vi "PixeLink MonitorAndSave.vi"(7 "Racine chemin de sauvegarde":path=path "G:/Développement de Programmes/Programmes/octo-labview/PixeLink - Homebrew/Data") -> ()   [LabVIEW 2014]
uses:
  <vilib>/addons/PixeLINK/Low Level Functions/ACQUISITION.llb/TDPU-Acquisition-StreamState.ctl
  <vilib>/addons/PixeLINK/Low Level Functions/CAMERA_FEATURES.llb/TDPU-CameraFeatures-FeatureIds.ctl
  <vilib>/addons/PixeLINK/Low Level Functions/CAMERA_FEATURES.llb/TDPU-CameraFeatures-FeatureFlags.ctl
  <vilib>/Platform/TimedLoop/XDataNode/timing_clust.ctl
  <vilib>/Platform/TimedLoop/XDataNode/nitl_modes.ctl
  <vilib>/Platform/TimedLoop/XDataNode/wakeup.ctl
  <vilib>/platform/TimedLoop/XDataNode/XDataNode.xnode
  <vilib>/Platform/TimedLoop/XDataNode/XDNodeRunTimeDep.lvlib
panel:
  out "Div":dbl
  out "Imager Serial #":u32[](array[numeric])
  in  "Chemins de sauvegarde":path[](array[path])
  in  "Bind Path to Camera":bool
  in  "Automatic\nfolder naming":bool=TRUE
  in  "Imager":u32(ring)=741003962 items=["Cam 0"=741003962]
  out "Error OUT 2":errorcluster
  out "Error OUT":errorcluster
  in  "Overwrite?":bool
  in  "Snap current Data":bool
  in  "Save Data":bool
  out "Warning":bool
  out "Message":string
  in  "Indice":u32
  in  "Nom du fichier":string="tir"
  in  "Mode de Sauvegarde":u16(ring)=1 items=["Manuel", "Automatique"]
  out "Captured Image":dbl[][](graph)
  out "Waiting for Trigger":bool
  in  "Continuous Grab":bool
  in  "Snap Next frame":bool
  out "Camera Handle":u32
  in  "Stop Grab\n(Insistez!)":bool
  in  "Trigger Type":enum16{"Free Running", "Software", "Hardware"}(ring)
  in  "Trigger Polarity":enum16{"Positive", "Negative"}(ring)
  in  "Refresh Trigger":bool
  in  "Exposure Time":dbl(slide) min=3.9999998989515007e-05 max=1.0 scale=3.9999998989515007e-05..1.0
  in  "stop":bool
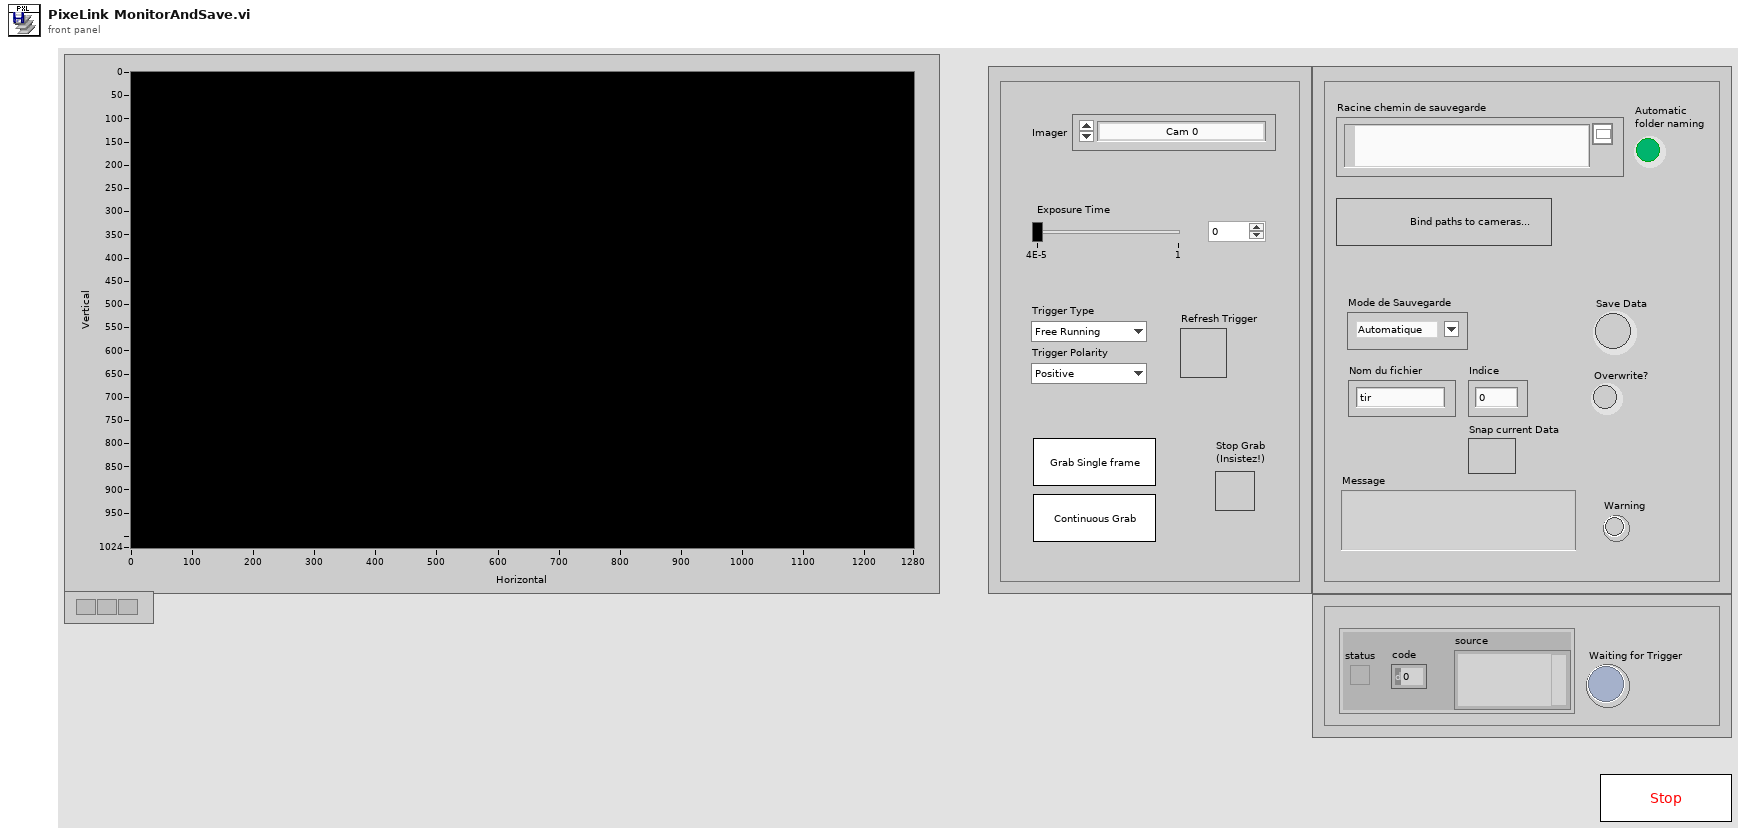
[diagram p1: front panel]
types:
  T1 = typedef "TDPU-Acquisition-StreamState.ctl" = u32
  T2 = typedef "TDPU-CameraFeatures-FeatureFlags.ctl" = u32
  T3 = typedef "TDPU-CameraFeatures-FeatureIds.ctl" = u32
  T4 = typedef "XDNodeRunTimeDep.lvlib/timing_clust.ctl" = cluster{"Expected End [f-1]":u64, "Actual End [f-1]":u64, "Finished Late? [f-1]":bool, "Expected End [i-1]":u64, "Actual End [i-1]":u64, "Finished Late? [i-1]":bool, "Expected Start [i]":u64, "Actual Start [i]":u64, "Expected Start [f]":u64, "Actual Start [f]":u64, "Source Name":string, "Structure Name":string, "Period":i64, "Deadline":i64, "Offset":i64, "Start":i64, "Priority":i32, "Timeout":i32, "Mode":T5, "Wakeup Reason":T6, "Error":errorcluster, "Source Type":string, "Secondary Source Type":string, "Global End Time":u64, "Global Start Time":u64, "Frame Duration":u64, "Iteration Duration":u64, "Assigned CPU":i32, "I/O Scan Engine Mode":u32}
  T5 = typedef "XDNodeRunTimeDep.lvlib/nitl_modes.ctl" = enum32{"No Change", "Process missed periods, maintain original phase", "Discard missed periods, maintain original phase", "Process missed periods, ignore original phase", "Discard missed periods, ignore original phase"}
  T6 = typedef "XDNodeRunTimeDep.lvlib/wakeup.ctl" = enum32{"Normal", "Aborted", "Asynchronous wakeup", "Timing source error", "Timed loop error", "Timeout"}
  T7 = typedef "LVStringsAndValuesArrayTypeDef_U32.ctl" = cluster{"String":string, "Value":u32}[]
  T8 = typedef "TDPU-Identification-Camera_Info.ctl" = cluster{"VendorName":string, "ModelName":string, "Description":string, "SerialNumber":string, "FirmwareVersion":string, "FPGAVersion":string, "CameraName":string}
  T9 = typedef "TDPU-Acquisition-Frame_Desc.ctl" = cluster{"uSize":u32, "fFrameTime":dbl, "uFrameNumber":u32, "Brightness":cluster{"fValue":dbl}, "AutoExposure":cluster{"fValue":dbl}, "Sharpness":cluster{"fValue":dbl}, "WhiteBalance":cluster{"fValue":dbl}, "Hue":cluster{"fValue":dbl}, "Saturation":cluster{"fValue":dbl}, "Gamma":cluster{"fValue":dbl}, "Shutter":cluster{"fValue":dbl}, "Gain":cluster{"fValue":dbl}, "Iris":cluster{"fValue":dbl}, "Focus":cluster{"fValue":dbl}, "Temperature":cluster{"fValue":dbl}, "Trigger":cluster{"fMode":dbl, "fType":dbl, "fPolarity":dbl, "fDelay":dbl, "fParameter":dbl}, "Zoom":cluster{"fValue":dbl}, "Pan":cluster{"fValue":dbl}, "Tilt":cluster{"fValue":dbl}, "OpticalFilter":cluster{"fValue":dbl}, "GPIO":cluster{"fMode":dbl[], "fPolarity":dbl[], "fParameter1":dbl[], "fParameter2":dbl[], "fParameter3":dbl[]}, "FrameRate":cluster{"fValue":dbl}, "ROI":cluster{"fLeft":dbl, "fTop":dbl, "fWidth":dbl, "fHeight":dbl}, "Flip":cluster{"fHorizontal":dbl, "fVertical":dbl}, "PixelAddressingValue":cluster{"fValue":dbl}, "PixelFormat":cluster{"fValue":dbl}, "ExtendedShutter":cluster{"fKneePoint":dbl[]}, "AutoROI":cluster{"fLeft":dbl, "fTop":dbl, "fWidth":dbl, "fHeight":dbl}, "WhiteShading":cluster{"fRedGain":dbl, "fGreenGain":dbl, "fBlueGain":dbl}, "Rotate":cluster{"fValue":dbl}, "PixelAddressingMode":cluster{"fValue":dbl}}
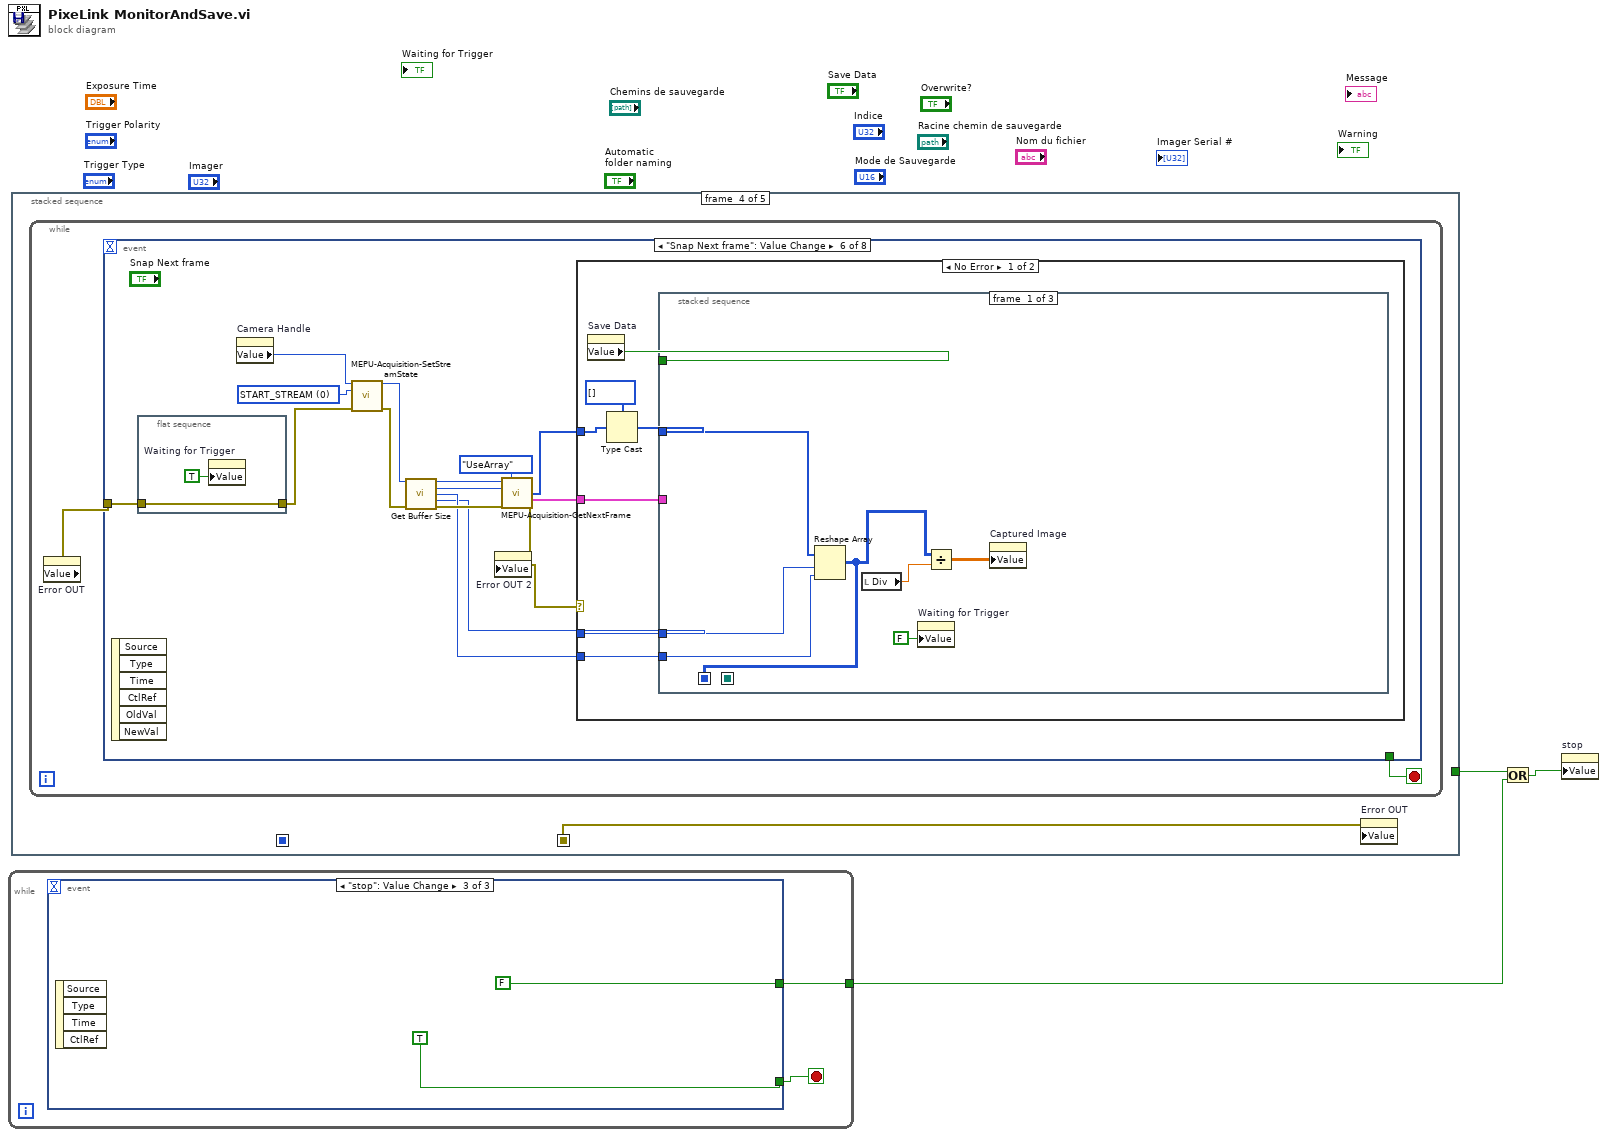
[diagram p0: block diagram]
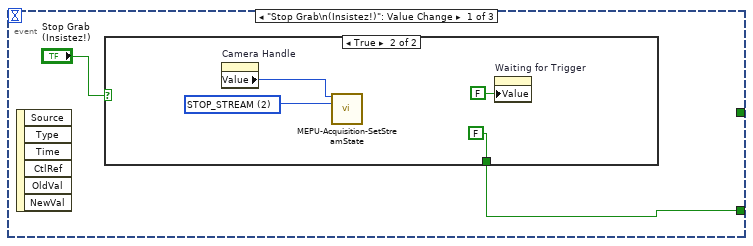
[diagram p2: hidden frame]
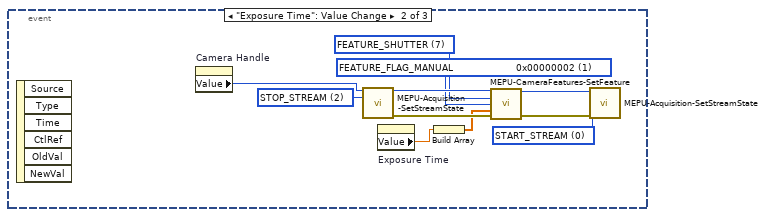
[diagram p4: hidden frame]
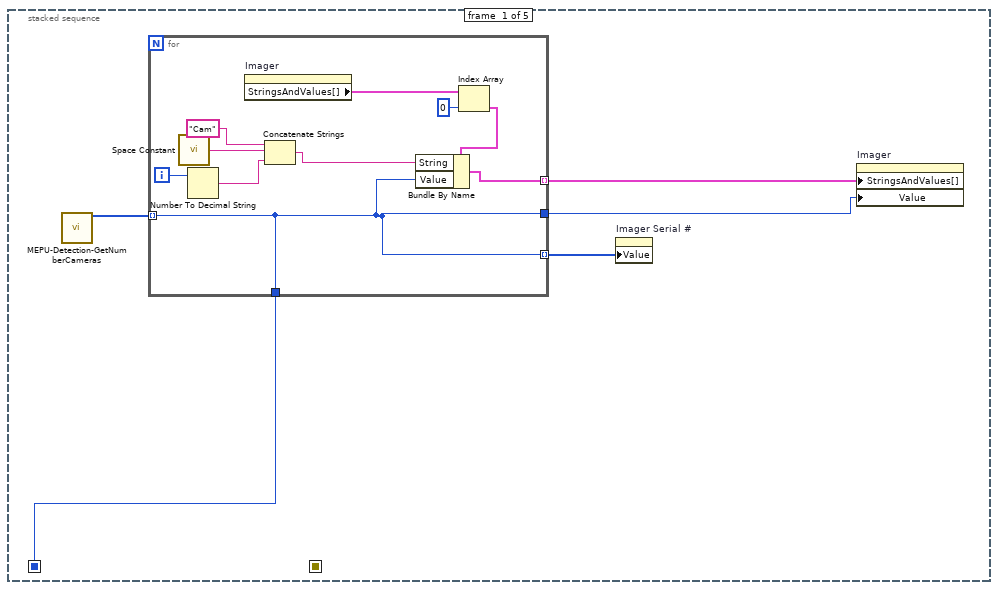
[diagram p5: hidden frame]
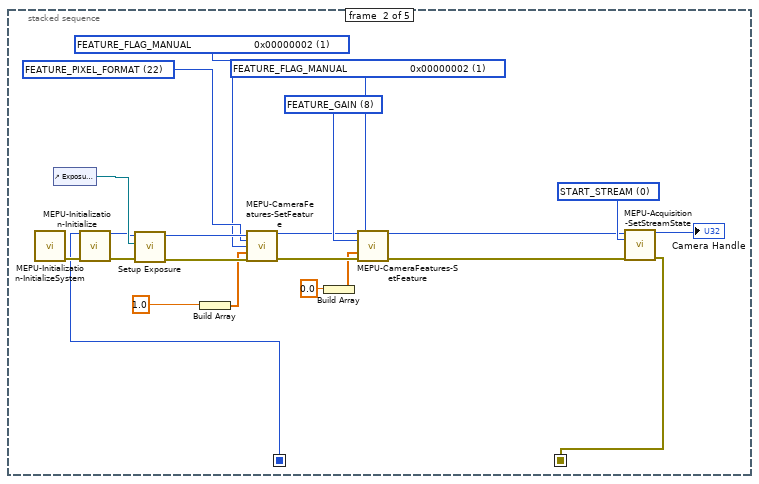
[diagram p6: hidden frame]
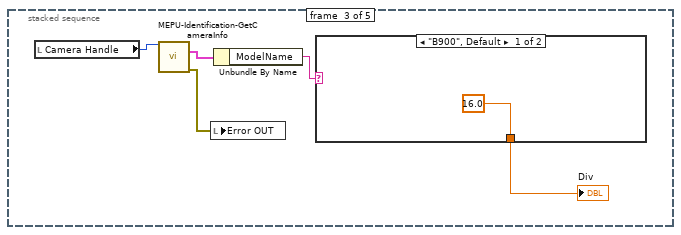
[diagram p7: hidden frame]
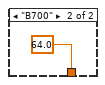
[diagram p8: hidden frame]
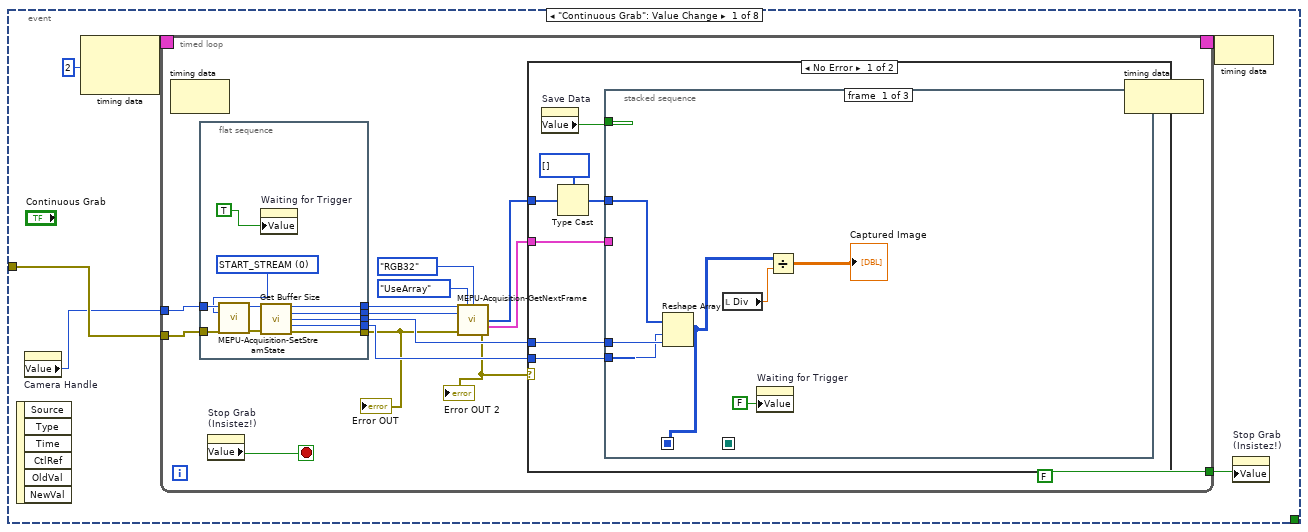
[diagram p9: hidden frame]
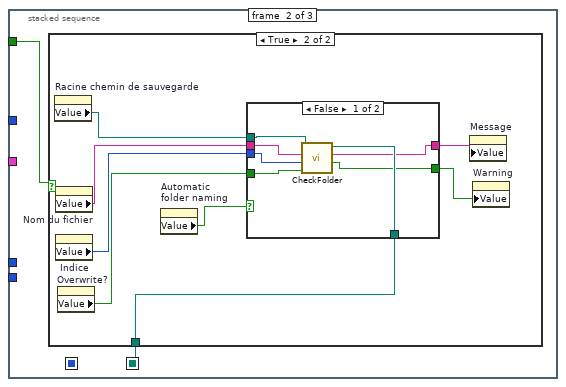
[diagram p10: hidden frame]
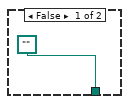
[diagram p11: hidden frame]
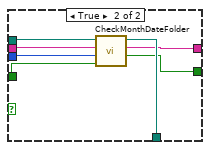
[diagram p12: hidden frame]
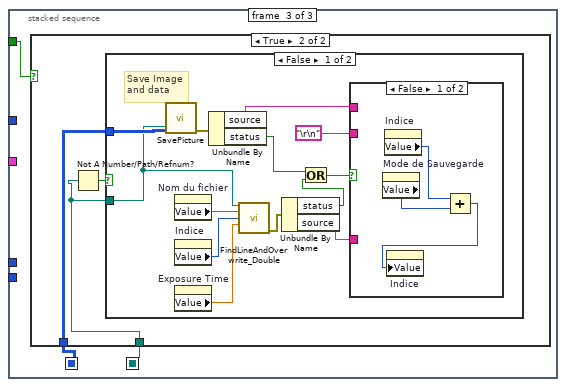
[diagram p13: hidden frame]
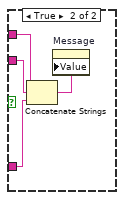
[diagram p15: hidden frame]
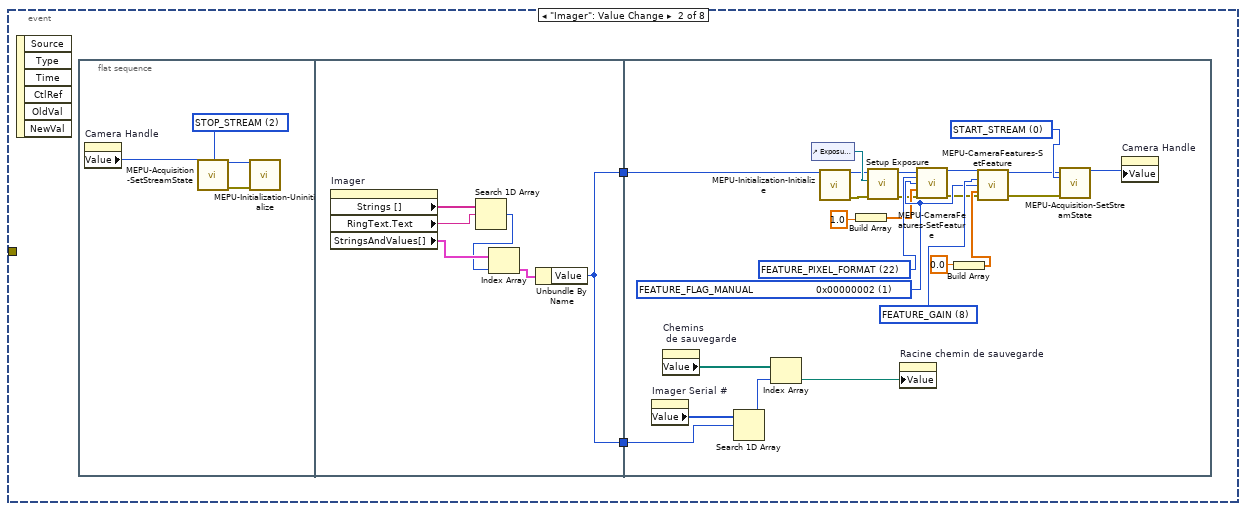
[diagram p18: hidden frame]
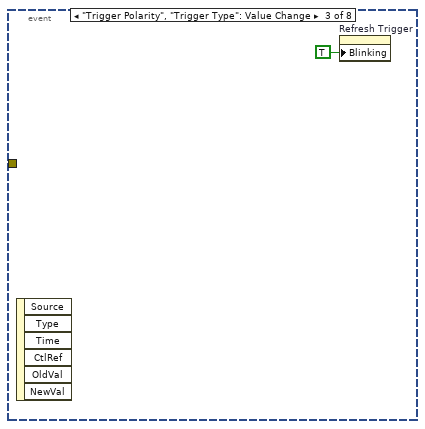
[diagram p19: hidden frame]
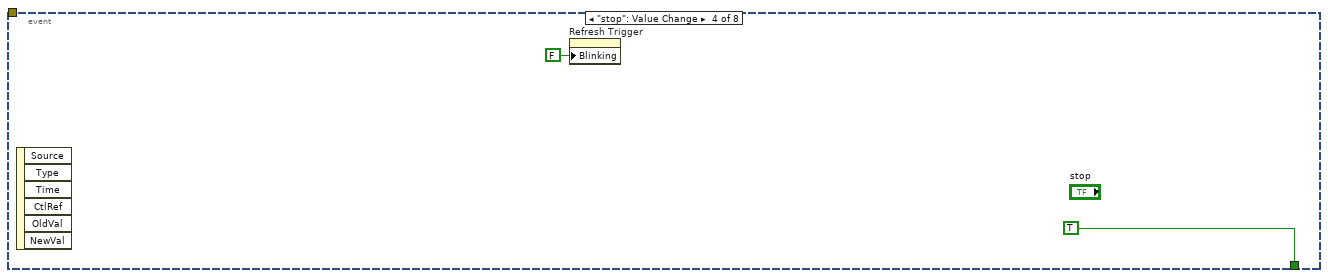
[diagram p20: hidden frame]
diagram:
  n1 = while {
    tunnel: [w4] -> w2
    stop <- w5 stop-if-true
    n2 = event shown="[2] \"stop\": Value Change" {
      selector: _ -> [_ _ _]
      dyn-events: _ -> [_ _ _]
      timeout: _ -> [_ _ _]
      tunnel: [w6 _ TRUE] -> w5
      tunnel: [_ _ FALSE] -> w4
      event "Stop Grab\n(Insistez!)": Value Change {
        n3 = event-data() -> ()  [unwired: 1 in, 6 out]
        n4 = case shown="True" "Stop Grab\n(Insistez!)" {
          tunnel: [_ FALSE] -> w6
          frame False {
          }
          frame True {
            w11 = T1 2 items=["START_STREAM", "PAUSE_STREAM", "STOP_STREAM"] ("uStreamState IN")
            n5 = property on="Camera Handle" class="DigNum (strict)"() -> ("Value"=w9:u32)  [unwired: 2 in, 2 out]
            n6 = call <vilib>:"MEPU-Acquisition-SetStreamState.vi"("hCamera IN"=w9, "uStreamState IN"=w11) -> ()  [unwired: 12 in, 2 out]
            n7 = property on="Waiting for Trigger" class="Bool (strict)"("Value"=FALSE ("Waiting for Trigger")) -> ()  [unwired: 2 in, 2 out]
          }
        }
      }
      event "Exposure Time": Value Change {
        w22 = T1 0 items=["START_STREAM", "PAUSE_STREAM", "STOP_STREAM"] ("uStreamState IN")
        w21 = T1 2 items=["START_STREAM", "PAUSE_STREAM", "STOP_STREAM"] ("uStreamState IN")
        w14 = T2 1 items=["FEATURE_FLAG_PRESENCE                 0x00000001", "FEATURE_FLAG_MANUAL                     0x00000002", "FEATURE_FLAG_AUTO                         0x00000004", "FEATURE_FLAG_ONEPUSH                   0x00000008", "FEATURE_FLAG_OFF                            0x00000010", "FEATURE_FLAG_DESC_SUPPORTED    0x00000020", "FEATURE_FLAG_READ_ONLY               0x00000040"] ("uFlags IN")
        w13 = T3 7 items=["FEATURE_BRIGHTNESS", "FEATURE_EXPOSURE", "FEATURE_SHARPNESS", "FEATURE_WHITE_BAL", "FEATURE_HUE", "FEATURE_SATURATION", "FEATURE_GAMMA", "FEATURE_SHUTTER", "FEATURE_GAIN", "FEATURE_IRIS", "FEATURE_FOCUS", "FEATURE_TEMPERATURE", "FEATURE_TRIGGER", "FEATURE_ZOOM", "FEATURE_PAN", "FEATURE_TILT", "FEATURE_OPT_FILTER", "FEATURE_GPIO", "FEATURE_FRAME_RATE", "FEATURE_ROI", "FEATURE_FLIP", "FEATURE_PIXEL_ADDRESSING", "FEATURE_PIXEL_FORMAT", "FEATURE_EXTENDED_SHUTTER", "FEATURE_AUTO_ROI", "FEATURE_LOOKUP_TABLE", "FEATURE_MEMORY_CHANNEL", "FEATURE_WHITE_SHADING", "FEATURE_ROTATE", "FEATURE_IMAGER_CLK_DIVISOR", "FEATURE_TRIG_WITH_CNTRLD_LIGHT", "FEATURE_MAX_PIXEL_SIZE"] ("uFeatureId IN")
        n8 = event-data() -> ()  [unwired: 1 in, 6 out]
        n9 = property on="Camera Handle" class="DigNum (strict)"() -> ("Value"=w12:u32)  [unwired: 2 in, 2 out]
        n10 = call <vilib>:"MEPU-Acquisition-SetStreamState.vi"("hCamera IN"=w12, "uStreamState IN"=w21) -> ("hCamera OUT"=w17:u32, "Error OUT"=w20:errorcluster)  [unwired: 12 in]
        n11 = property on="Exposure Time" class="Slide (strict)"() -> ("Value"=w15:dbl)  [unwired: 2 in, 2 out]
        n12 = Build Array(w15) -> (w16:dbl[])
        n13 = call <vilib>:"MEPU-CameraFeatures-SetFeature.vi"("hCamera IN"=w17, "uFeatureId IN"=w13, "uFlags IN"=w14, "pParms IN"=w16, "Error IN"=w20) -> ("hCamera OUT"=w18:u32, "Error OUT"=w19:errorcluster)  [unwired: 9 out]
        n14 = call <vilib>:"MEPU-Acquisition-SetStreamState.vi"("hCamera IN"=w18, "uStreamState IN"=w22, "Error IN"=w19) -> ()  [unwired: 11 in, 2 out]
      }
      event "stop": Value Change {
        n15 = event-data() -> ()  [unwired: 1 in, 4 out]
      }
    }
  }
  n16 = stacked-sequence {
    seq-local: [_ w50 _ _ _] -> [_ _ _ w69 _]
    seq-local: [w28 _ _ _ _] -> [_ w40 _ _ _]
    tunnel: [_ _ _ _ TRUE] -> w3
    frame #0 {
      n17 = call <vilib>:"MEPU-Detection-GetNumberCameras.vi"() -> ("LV_SerialNumbers OUT"=w29:u32[])  [unwired: 13 in, 2 out]
      n18 = for {
        tunnel: w29 -> [w30] mode=indexing
        tunnel: [w34] -> w27 mode=indexing
        tunnel: [w30] -> w28
        tunnel: [w30] -> w26
        tunnel: [w30] -> w25 mode=indexing
        i -> [w39]
        n19 = call <vilib>:"Space Constant.vi"() -> ("String"=w37:string)
        n20 = Number To Decimal String(number=w39) -> (decimal integer string=w36:string)  [unwired: 1 in]
        n21 = property on="Imager" class="Ring (strict)"() -> ("StringsAndValues[]"=w33:T7)  [unwired: 2 in, 2 out]
        n22 = Concatenate Strings("Cam", w37, w36) -> (w35:string)
        n23 = Index Array(array=w33, index=0) -> (element=w31:cluster{"String":string, "Value":u32})
        n24 = Bundle By Name(cluster=w31, "String"=w35, "Value"=w30) -> (w34:cluster{"String":string, "Value":u32})
      }
      n25 = property on="Imager Serial #" class="Arr (strict)"("Value"=w25) -> ()  [unwired: 2 in, 2 out]
      n26 = property on="Imager" class="Ring (strict)"("StringsAndValues[]"=w27, "Value"=w26) -> ()  [unwired: 2 in, 2 out]
    }
    frame #1 {
      w45 = T2 1 items=["FEATURE_FLAG_PRESENCE                 0x00000001", "FEATURE_FLAG_MANUAL                     0x00000002", "FEATURE_FLAG_AUTO                         0x00000004", "FEATURE_FLAG_ONEPUSH                   0x00000008", "FEATURE_FLAG_OFF                            0x00000010", "FEATURE_FLAG_DESC_SUPPORTED    0x00000020", "FEATURE_FLAG_READ_ONLY               0x00000040"] ("uFlags IN")
      w44 = T3 8 items=["FEATURE_BRIGHTNESS", "FEATURE_EXPOSURE", "FEATURE_SHARPNESS", "FEATURE_WHITE_BAL", "FEATURE_HUE", "FEATURE_SATURATION", "FEATURE_GAMMA", "FEATURE_SHUTTER", "FEATURE_GAIN", "FEATURE_IRIS", "FEATURE_FOCUS", "FEATURE_TEMPERATURE", "FEATURE_TRIGGER", "FEATURE_ZOOM", "FEATURE_PAN", "FEATURE_TILT", "FEATURE_OPT_FILTER", "FEATURE_GPIO", "FEATURE_FRAME_RATE", "FEATURE_ROI", "FEATURE_FLIP", "FEATURE_PIXEL_ADDRESSING", "FEATURE_PIXEL_FORMAT", "FEATURE_EXTENDED_SHUTTER", "FEATURE_AUTO_ROI", "FEATURE_LOOKUP_TABLE", "FEATURE_MEMORY_CHANNEL", "FEATURE_WHITE_SHADING", "FEATURE_ROTATE", "FEATURE_IMAGER_CLK_DIVISOR", "FEATURE_TRIG_WITH_CNTRLD_LIGHT", "FEATURE_MAX_PIXEL_SIZE"] ("uFeatureId IN")
      w53 = T2 1 items=["FEATURE_FLAG_PRESENCE                 0x00000001", "FEATURE_FLAG_MANUAL                     0x00000002", "FEATURE_FLAG_AUTO                         0x00000004", "FEATURE_FLAG_ONEPUSH                   0x00000008", "FEATURE_FLAG_OFF                            0x00000010", "FEATURE_FLAG_DESC_SUPPORTED    0x00000020", "FEATURE_FLAG_READ_ONLY               0x00000040"] ("uFlags IN")
      w54 = T3 22 items=["FEATURE_BRIGHTNESS", "FEATURE_EXPOSURE", "FEATURE_SHARPNESS", "FEATURE_WHITE_BAL", "FEATURE_HUE", "FEATURE_SATURATION", "FEATURE_GAMMA", "FEATURE_SHUTTER", "FEATURE_GAIN", "FEATURE_IRIS", "FEATURE_FOCUS", "FEATURE_TEMPERATURE", "FEATURE_TRIGGER", "FEATURE_ZOOM", "FEATURE_PAN", "FEATURE_TILT", "FEATURE_OPT_FILTER", "FEATURE_GPIO", "FEATURE_FRAME_RATE", "FEATURE_ROI", "FEATURE_FLIP", "FEATURE_PIXEL_ADDRESSING", "FEATURE_PIXEL_FORMAT", "FEATURE_EXTENDED_SHUTTER", "FEATURE_AUTO_ROI", "FEATURE_LOOKUP_TABLE", "FEATURE_MEMORY_CHANNEL", "FEATURE_WHITE_SHADING", "FEATURE_ROTATE", "FEATURE_IMAGER_CLK_DIVISOR", "FEATURE_TRIG_WITH_CNTRLD_LIGHT", "FEATURE_MAX_PIXEL_SIZE"] ("uFeatureId IN")
      w60 = T1 0 items=["START_STREAM", "PAUSE_STREAM", "STOP_STREAM"] ("uStreamState IN")
      n27 = call <vilib>:"MEPU-Initialization-InitializeSystem.vi"() -> ("Error OUT"=w61:errorcluster)  [unwired: 15 in]
      n28 = control-ref of="Exposure Time"() -> (w59:refnum<vi>)
      n29 = call <vilib>:"MEPU-Initialization-Initialize.vi"("uSerialNumber IN"=w40, "Error IN"=w61) -> ("phCamera OUT"=w58:u32, "Error OUT"=w57:errorcluster)  [unwired: 11 in, 1 out]
      n30 = call "Setup Exposure.vi"("Error IN"=w57, "Shutter"=w59, "hCamera IN"=w58) -> ("Error OUT"=w56:errorcluster, "phCamera OUT"=w55:u32)  [unwired: 7 in]
      n31 = Build Array(1.0) -> (w51:dbl[])
      n32 = call <vilib>:"MEPU-CameraFeatures-SetFeature.vi"("hCamera IN"=w55, "uFeatureId IN"=w54, "uFlags IN"=w53, "pParms IN"=w51, "Error IN"=w56) -> ("hCamera OUT"=w43:u32, "Error OUT"=w48:errorcluster)  [unwired: 8 in, 1 out]
      n33 = Build Array(0.0) -> (w46:dbl[])
      n34 = call <vilib>:"MEPU-CameraFeatures-SetFeature.vi"("hCamera IN"=w43, "uFeatureId IN"=w44, "uFlags IN"=w45, "pParms IN"=w46, "Error IN"=w48) -> ("hCamera OUT"=w42:u32, "Error OUT"=w41:errorcluster)  [unwired: 8 in, 1 out]
      n35 = call <vilib>:"MEPU-Acquisition-SetStreamState.vi"("hCamera IN"=w42, "uStreamState IN"=w60, "Error IN"=w41) -> ("hCamera OUT"=→"Camera Handle":u32, "Error OUT"=w50:errorcluster)  [unwired: 11 in]
    }
    frame #2 {
      n36 = local read "Camera Handle"() -> (w66:u32)
      n37 = call <vilib>:"MEPU-Identification-GetCameraInfo.vi"("hCamera IN"=w66) -> ("pLVCameraInfo OUT"=w65:T8, "Error OUT"=w62:errorcluster)  [unwired: 12 in, 1 out]
      n38 = local write "Error OUT"(w62) -> ()
      n39 = Unbundle By Name(w65) -> ("ModelName"=w64:string)
      n40 = case shown="\"B900\", Default" w64 {
        tunnel: [16.0 64.0] -> w63
        frame "B900", Default {
        }
        frame "B700" {
        }
      }
      "Div" <- w63
    }
    frame #3 {
      n41 = while {
        stop <- w71 stop-if-true
        n42 = property on="Error OUT" class="Clust (strict)"() -> ("Value"=w70:errorcluster)  [unwired: 2 in, 2 out]
        n43 = event shown="[5] \"Snap Next frame\": Value Change" {
          selector: _ -> [_ _ _ _ _ _ _ _]
          dyn-events: _ -> [_ _ _ _ _ _ _ _]
          timeout: _ -> [_ _ _ _ _ _ _ _]
          tunnel: w70 -> [w77 _ _ _ w221 w239 _ _]
          tunnel: [_ _ _ TRUE _ _ _ _] -> w71
          event "Continuous Grab": Value Change {
            n44 = event-data() -> ()  [unwired: 1 in, 6 out]
            n45 = property on="Camera Handle" class="DigNum (strict)"() -> ("Value"=w72:u32)  [unwired: 2 in, 2 out]
            n46 = node-c288(i64 2 ("Period")) -> (w76:T4)  [unwired: 1 in]
            n47 = timed-loop {
              timing: w76 -> [_]
              timing-out: [_] -> w75
              tunnel: w72 -> [w91]
              tunnel: w77 -> [w85]
              tunnel: [FALSE] -> w73
              stop <- w82 stop-if-true
              n48 = node-c288() -> ()  [unwired: 1 in, 1 out]
              n49 = flat-sequence {
                tunnel: w91 -> [w158]
                tunnel: [w167] -> w90
                tunnel: [w166] -> w89
                tunnel: [w165] -> w80
                tunnel: w85 -> [w161]
                tunnel: [w164] -> w84
                tunnel: [w163] -> w83
                frame #0 {
                  w157 = T1 0 items=["START_STREAM", "PAUSE_STREAM", "STOP_STREAM"] ("uStreamState IN")
                  n50 = call <vilib>:"MEPU-Acquisition-SetStreamState.vi"("hCamera IN"=w158, "uStreamState IN"=w157, "Error IN"=w161) -> ("hCamera OUT"=w159:u32, "Error OUT"=w160:errorcluster)  [unwired: 11 in]
                  n51 = property on="Waiting for Trigger" class="Bool (strict)"("Value"=TRUE ("Waiting for Trigger")) -> ()  [unwired: 2 in, 2 out]
                  n52 = call "Get Buffer Size.vi"("phCamera IN"=w159, "Error IN"=w160) -> ("phCamera OUT"=w167:u32, "uBufferSize OUT"=w166:u32, "uWidth OUT"=w164:u32, "uHeight OUT"=w163:u32, "Error OUT"=w165:errorcluster)  [unwired: 8 in, 1 out]
                }
              }
              n53 = property on="Stop Grab\n(Insistez!)" class="Bool (strict)"() -> ("Value"=w82:bool)  [unwired: 2 in, 2 out]
              n54 = call <vilib>:"MEPU-Acquisition-GetNextFrame.vi"("hCamera IN"=w90, "Mode IN"=enum16{"UseArray", "UsePointer"}."UseArray", "OutputMode IN"=enum16{"Default", "RGB24", "RGB32"}."RGB32", "uBufferSize IN"=w89, "Error IN"=w80) -> ("Data OUT"=w86:u8[], "pDescriptor"=w78:T9, "Error OUT"=w79:errorcluster)  [unwired: 6 in, 2 out]
              "Error OUT 2" <- w79
              n55 = case shown="No Error" w79 {
                tunnel: w86 -> [w98 _]
                tunnel: w84 -> [w95 _]
                tunnel: w83 -> [w94 _]
                tunnel: w78 -> [w92 _]
                frame No Error {
                  n56 = property on="Save Data" class="Bool (strict)"() -> ("Value"=w93:bool)  [unwired: 2 in, 2 out]
                  n57 = Type Cast(type=u16[] [] ("Data OUT"), x=w98) -> (*(type *) &x=w96:u16[])
                  n58 = stacked-sequence {
                    seq-local: [_ w107 _] -> [_ _ w133]
                    seq-local: [w101 _ _] -> [_ _ w131]
                    tunnel: w96 -> [w105 _ _]
                    tunnel: w95 -> [w104 _ _]
                    tunnel: w94 -> [w103 _ _]
                    tunnel: w93 -> [_ w106 w132]
                    tunnel: w92 -> [_ _ _]
                    frame #0 {
                      n59 = Reshape Array(w105, w103, w104) -> (w101:u16[][])
                      n60 = local read "Div"() -> (w100:dbl)
                      n61 = property on="Waiting for Trigger" class="Bool (strict)"("Value"=FALSE ("Waiting for Trigger")) -> ()  [unwired: 2 in, 2 out]
                      n62 = Divide(x=w101, y=w100) -> (x/y=→"Captured Image":dbl[][])
                    }
                    frame #1 {
                      n63 = case shown="True" w106 {
                        tunnel: [path "" ("File Path") w112] -> w107
                        frame False {
                        }
                        frame True {
                          n64 = property on="Racine chemin de sauvegarde" class="Path"() -> ("Value"=w113:path)  [unwired: 2 in, 2 out]
                          n65 = property on="Nom du fichier" class="Str"() -> ("Value"=w114:string)  [unwired: 2 in, 2 out]
                          n66 = property on="Indice" class="DigNum (strict)"() -> ("Value"=w115:u32)  [unwired: 2 in, 2 out]
                          n67 = property on="Overwrite?" class="Bool (strict)"() -> ("Value"=w116:bool)  [unwired: 2 in, 2 out]
                          n68 = property on="Automatic\nfolder naming" class="Bool (strict)"() -> ("Value"=w109:bool)  [unwired: 2 in, 2 out]
                          n69 = case shown="False" w109 {
                            tunnel: w116 -> [w121 w130]
                            tunnel: w115 -> [w122 w129]
                            tunnel: w114 -> [w123 w128]
                            tunnel: w113 -> [w120 w127]
                            tunnel: [w119 w126] -> w112
                            tunnel: [w118 w125] -> w111
                            tunnel: [w117 w124] -> w110
                            frame False {
                              n70 = call "CheckFolder.vi"("Overwrite?"=w121, "Index"=w122, "File Name"=w123, "Folder Path Control"=w120) -> ("Warning"=w117:bool, "Message"=w118:string, "File Path"=w119:path)  [unwired: 5 in]
                            }
                            frame True {
                              n71 = call "CheckMonthDateFolder.vi"("Overwrite?"=w130, "Index"=w129, "File Name"=w128, "Folder Path Control"=w127) -> ("Warning"=w124:bool, "Message"=w125:string, "File Path"=w126:path)  [unwired: 5 in]
                            }
                          }
                          n72 = property on="Message" class="Str"("Value"=w111) -> ()  [unwired: 2 in, 2 out]
                          n73 = property on="Warning" class="Bool (strict)"("Value"=w110) -> ()  [unwired: 2 in, 2 out]
                        }
                      }
                    }
                    frame #2 {
                      n74 = case shown="True" w132 {
                        tunnel: w133 -> [_ w135]
                        tunnel: w131 -> [_ w134]
                        frame False {
                        }
                        frame True {
                          n75 = Not A Number/Path/Refnum?(number/path/refnum=w135) -> (NaN/Path/Refnum?=w136:bool)
                          n76 = case shown="False" w136 {
                            tunnel: w135 -> [w140 _]
                            tunnel: w134 -> [w142 _]
                            frame False {
                              # "Save Image\nand data"
                              n77 = call "SavePicture.vi"("File Path"=w140, "Image Pixels (U16)"=w142) -> ("error out"=w148:errorcluster)  [unwired: 9 in]
                              n78 = property on="Nom du fichier" class="Str"() -> ("Value"=w139:string)  [unwired: 2 in, 2 out]
                              n79 = property on="Indice" class="DigNum (strict)"() -> ("Value"=w138:u32)  [unwired: 2 in, 2 out]
                              n80 = property on="Exposure Time" class="Slide (strict)"() -> ("Value"=w137:dbl)  [unwired: 2 in, 2 out]
                              n81 = Unbundle By Name(w148) -> ("source"=w145:string, "status"=w146:bool)
                              n82 = call "FindLineAndOverwrite_Double.vi"("Exposure path"=w140, "Name"=w139, "Index"=w138, "Exposure"=w137) -> ("error out"=w141:errorcluster)  [unwired: 11 in]
                              n83 = Unbundle By Name(w141) -> ("status"=w147:bool, "source"=w149:string)
                              n84 = Or(x=w146, y=w147) -> (x .or. y?=w144:bool)
                              n85 = case shown="False" w144 {
                                tunnel: w149 -> [_ w153]
                                tunnel: w145 -> [_ w156]
                                tunnel: "\r\n" -> [_ w154]
                                frame False {
                                n86 = property on="Mode de Sauvegarde" class="Ring (strict)"() -> ("Value"=w151:u16)  [unwired: 2 in, 2 out]
                                n87 = property on="Indice" class="DigNum (strict)"() -> ("Value"=w152:u32)  [unwired: 2 in, 2 out]
                                n88 = Add(x=w152, y=w151) -> (x+y=w150:u32)
                                n89 = property on="Indice" class="DigNum (strict)"("Value"=w150) -> ()  [unwired: 2 in, 2 out]
                                }
                                frame True {
                                n90 = Concatenate Strings(w156, w154, w153) -> (w155:string)
                                n91 = property on="Message" class="Str"("Value"=w155) -> ()  [unwired: 2 in, 2 out]
                                }
                              }
                            }
                            frame True {
                            }
                          }
                        }
                      }
                    }
                  }
                }
                frame Error {
                }
              }
              n92 = node-c288() -> ()  [unwired: 1 in, 1 out]
              "Error OUT" <- w80
            }
            n93 = node-c288(w75) -> ()
            n94 = property on="Stop Grab\n(Insistez!)" class="Bool (strict)"("Value"=w73) -> ()  [unwired: 2 in, 2 out]
          }
          event "Imager": Value Change {
            n95 = event-data() -> ()  [unwired: 1 in, 6 out]
            n96 = flat-sequence {
              tunnel: [w180] -> w175
              tunnel: [w180] -> w174
              tunnel: w175 -> [w191]
              tunnel: w174 -> [w187]
              frame #0 {
                w177 = T1 2 items=["START_STREAM", "PAUSE_STREAM", "STOP_STREAM"] ("uStreamState IN")
                n97 = property on="Camera Handle" class="DigNum (strict)"() -> ("Value"=w176:u32)  [unwired: 2 in, 2 out]
                n98 = call <vilib>:"MEPU-Acquisition-SetStreamState.vi"("hCamera IN"=w176, "uStreamState IN"=w177) -> ("hCamera OUT"=w178:u32, "Error OUT"=w179:errorcluster)  [unwired: 12 in]
                n99 = call <vilib>:"MEPU-Initialization-Uninitialize.vi"("hCamera IN"=w178, "Error IN"=w179) -> ()  [unwired: 13 in, 1 out]
              }
              frame #1 {
                n100 = property on="Imager" class="Ring (strict)"() -> ("Strings []"=w185:string[], "RingText.Text"=w184:string, "StringsAndValues[]"=w183:T7)  [unwired: 2 in, 2 out]
                n101 = Search 1D Array(1D array=w185, element=w184) -> (index of element=w182:i32)  [unwired: 1 in]
                n102 = Index Array(array=w183, index=w182) -> (element=w181:cluster{"String":string, "Value":u32})
                n103 = Unbundle By Name(w181) -> ("Value"=w180:u32)
              }
              frame #2 {
                w208 = T1 0 items=["START_STREAM", "PAUSE_STREAM", "STOP_STREAM"] ("uStreamState IN")
                w205 = T3 8 items=["FEATURE_BRIGHTNESS", "FEATURE_EXPOSURE", "FEATURE_SHARPNESS", "FEATURE_WHITE_BAL", "FEATURE_HUE", "FEATURE_SATURATION", "FEATURE_GAMMA", "FEATURE_SHUTTER", "FEATURE_GAIN", "FEATURE_IRIS", "FEATURE_FOCUS", "FEATURE_TEMPERATURE", "FEATURE_TRIGGER", "FEATURE_ZOOM", "FEATURE_PAN", "FEATURE_TILT", "FEATURE_OPT_FILTER", "FEATURE_GPIO", "FEATURE_FRAME_RATE", "FEATURE_ROI", "FEATURE_FLIP", "FEATURE_PIXEL_ADDRESSING", "FEATURE_PIXEL_FORMAT", "FEATURE_EXTENDED_SHUTTER", "FEATURE_AUTO_ROI", "FEATURE_LOOKUP_TABLE", "FEATURE_MEMORY_CHANNEL", "FEATURE_WHITE_SHADING", "FEATURE_ROTATE", "FEATURE_IMAGER_CLK_DIVISOR", "FEATURE_TRIG_WITH_CNTRLD_LIGHT", "FEATURE_MAX_PIXEL_SIZE"] ("uFeatureId IN")
                w204 = T2 1 items=["FEATURE_FLAG_PRESENCE                 0x00000001", "FEATURE_FLAG_MANUAL                     0x00000002", "FEATURE_FLAG_AUTO                         0x00000004", "FEATURE_FLAG_ONEPUSH                   0x00000008", "FEATURE_FLAG_OFF                            0x00000010", "FEATURE_FLAG_DESC_SUPPORTED    0x00000020", "FEATURE_FLAG_READ_ONLY               0x00000040"] ("uFlags IN")
                w199 = T3 22 items=["FEATURE_BRIGHTNESS", "FEATURE_EXPOSURE", "FEATURE_SHARPNESS", "FEATURE_WHITE_BAL", "FEATURE_HUE", "FEATURE_SATURATION", "FEATURE_GAMMA", "FEATURE_SHUTTER", "FEATURE_GAIN", "FEATURE_IRIS", "FEATURE_FOCUS", "FEATURE_TEMPERATURE", "FEATURE_TRIGGER", "FEATURE_ZOOM", "FEATURE_PAN", "FEATURE_TILT", "FEATURE_OPT_FILTER", "FEATURE_GPIO", "FEATURE_FRAME_RATE", "FEATURE_ROI", "FEATURE_FLIP", "FEATURE_PIXEL_ADDRESSING", "FEATURE_PIXEL_FORMAT", "FEATURE_EXTENDED_SHUTTER", "FEATURE_AUTO_ROI", "FEATURE_LOOKUP_TABLE", "FEATURE_MEMORY_CHANNEL", "FEATURE_WHITE_SHADING", "FEATURE_ROTATE", "FEATURE_IMAGER_CLK_DIVISOR", "FEATURE_TRIG_WITH_CNTRLD_LIGHT", "FEATURE_MAX_PIXEL_SIZE"] ("uFeatureId IN")
                n104 = property on="Imager Serial #" class="Arr (strict)"() -> ("Value"=w188:u32[])  [unwired: 2 in, 2 out]
                n105 = property on="Chemins\n de sauvegarde" class="Arr (strict)"() -> ("Value"=w190:path[])  [unwired: 2 in, 2 out]
                n106 = Search 1D Array(1D array=w188, element=w187) -> (index of element=w186:i32)  [unwired: 1 in]
                n107 = Index Array(array=w190, index=w186) -> (element=w189:path)
                n108 = control-ref of="Exposure Time"() -> (w194:refnum<vi>)
                n109 = call <vilib>:"MEPU-Initialization-Initialize.vi"("uSerialNumber IN"=w191) -> ("phCamera OUT"=w193:u32, "Error OUT"=w192:errorcluster)  [unwired: 12 in, 1 out]
                n110 = Build Array(1.0) -> (w198:dbl[])
                n111 = call "Setup Exposure.vi"("Error IN"=w192, "Shutter"=w194, "hCamera IN"=w193) -> ("Error OUT"=w196:errorcluster, "phCamera OUT"=w195:u32)  [unwired: 7 in]
                n112 = property on="Racine chemin de sauvegarde" class="Path"("Value"=w189) -> ()  [unwired: 2 in, 2 out]
                n113 = call <vilib>:"MEPU-CameraFeatures-SetFeature.vi"("hCamera IN"=w195, "uFeatureId IN"=w199, "uFlags IN"=w204, "pParms IN"=w198, "Error IN"=w196) -> ("hCamera OUT"=w200:u32, "Error OUT"=w201:errorcluster)  [unwired: 8 in, 1 out]
                n114 = Build Array(0.0) -> (w203:dbl[])
                n115 = call <vilib>:"MEPU-CameraFeatures-SetFeature.vi"("hCamera IN"=w200, "uFeatureId IN"=w205, "uFlags IN"=w204, "pParms IN"=w203, "Error IN"=w201) -> ("hCamera OUT"=w206:u32, "Error OUT"=w207:errorcluster)  [unwired: 8 in, 1 out]
                n116 = call <vilib>:"MEPU-Acquisition-SetStreamState.vi"("hCamera IN"=w206, "uStreamState IN"=w208, "Error IN"=w207) -> ("hCamera OUT"=w209:u32)  [unwired: 11 in, 1 out]
                n117 = property on="Camera Handle" class="DigNum (strict)"("Value"=w209) -> ()  [unwired: 2 in, 2 out]
              }
            }
          }
          event "Trigger Polarity", "Trigger Type": Value Change {
            n118 = event-data() -> ()  [unwired: 1 in, 6 out]
            n119 = property on="Refresh Trigger" class="Bool"("Blinking"=TRUE) -> ()  [unwired: 2 in, 2 out]
          }
          event "stop": Value Change {
            n120 = event-data() -> ()  [unwired: 1 in, 6 out]
            n121 = property on="Refresh Trigger" class="Bool"("Blinking"=FALSE) -> ()  [unwired: 2 in, 2 out]
          }
          event "Refresh Trigger": Value Change {
            w215 = T1 2 items=["START_STREAM", "PAUSE_STREAM", "STOP_STREAM"] ("uStreamState IN")
            w216 = T1 0 items=["START_STREAM", "PAUSE_STREAM", "STOP_STREAM"] ("uStreamState IN")
            w230 = T2 1 items=["FEATURE_FLAG_PRESENCE                 0x00000001", "FEATURE_FLAG_MANUAL                     0x00000002", "FEATURE_FLAG_AUTO                         0x00000004", "FEATURE_FLAG_ONEPUSH                   0x00000008", "FEATURE_FLAG_OFF                            0x00000010", "FEATURE_FLAG_DESC_SUPPORTED    0x00000020", "FEATURE_FLAG_READ_ONLY               0x00000040"] ("uFlags IN")
            w231 = T3 12 items=["FEATURE_BRIGHTNESS", "FEATURE_EXPOSURE", "FEATURE_SHARPNESS", "FEATURE_WHITE_BAL", "FEATURE_HUE", "FEATURE_SATURATION", "FEATURE_GAMMA", "FEATURE_SHUTTER", "FEATURE_GAIN", "FEATURE_IRIS", "FEATURE_FOCUS", "FEATURE_TEMPERATURE", "FEATURE_TRIGGER", "FEATURE_ZOOM", "FEATURE_PAN", "FEATURE_TILT", "FEATURE_OPT_FILTER", "FEATURE_GPIO", "FEATURE_FRAME_RATE", "FEATURE_ROI", "FEATURE_FLIP", "FEATURE_PIXEL_ADDRESSING", "FEATURE_PIXEL_FORMAT", "FEATURE_EXTENDED_SHUTTER", "FEATURE_AUTO_ROI", "FEATURE_LOOKUP_TABLE", "FEATURE_MEMORY_CHANNEL", "FEATURE_WHITE_SHADING", "FEATURE_ROTATE", "FEATURE_IMAGER_CLK_DIVISOR", "FEATURE_TRIG_WITH_CNTRLD_LIGHT", "FEATURE_MAX_PIXEL_SIZE"] ("uFeatureId IN")
            n122 = event-data() -> ()  [unwired: 1 in, 6 out]
            n123 = property on="Camera Handle" class="DigNum (strict)"() -> ("Value"=w213:u32)  [unwired: 2 in, 2 out]
            n124 = property on="Refresh Trigger" class="Bool"("Blinking"=FALSE) -> ()  [unwired: 2 in, 2 out]
            n125 = property on="Trigger Polarity" class="Enum (strict)"() -> ("Value"=w226:enum16{"Positive", "Negative"})  [unwired: 2 in, 2 out]
            n126 = property on="Trigger Type" class="Enum (strict)"() -> ("Value"=w228:enum16{"Free Running", "Software", "Hardware"})  [unwired: 2 in, 2 out]
            n127 = To Double Precision Float(number=w226) -> (double precision float=w225:dbl)
            n128 = To Double Precision Float(number=w228) -> (double precision float=w227:dbl)
            n129 = Build Array(0.0 ("element"), w227, w225, 0.0 ("element"), 0.0 ("element")) -> (w222:dbl[])
            n130 = call <vilib>:"MEPU-Acquisition-SetStreamState.vi"("hCamera IN"=w213, "uStreamState IN"=w215, "Error IN"=w221) -> ("hCamera OUT"=w220:u32, "Error OUT"=w219:errorcluster)  [unwired: 11 in]
            n131 = call <vilib>:"MEPU-CameraFeatures-SetFeature.vi"("hCamera IN"=w220, "uFeatureId IN"=w231, "uFlags IN"=w230, "pParms IN"=w222, "Error IN"=w219) -> ("hCamera OUT"=w217:u32, "Error OUT"=w218:errorcluster)  [unwired: 9 out]
            n132 = call <vilib>:"MEPU-Acquisition-SetStreamState.vi"("hCamera IN"=w217, "uStreamState IN"=w216, "Error IN"=w218) -> ()  [unwired: 11 in, 2 out]
          }
          event "Snap Next frame": Value Change {
            w242 = T1 0 items=["START_STREAM", "PAUSE_STREAM", "STOP_STREAM"] ("uStreamState IN")
            n133 = event-data() -> ()  [unwired: 1 in, 6 out]
            n134 = flat-sequence {
              tunnel: w239 -> [w307]
              tunnel: [w307] -> w238
              frame #0 {
                n135 = property on="Waiting for Trigger" class="Bool (strict)"("Value"=TRUE ("Waiting for Trigger")) -> ()  [unwired: 2 in, 2 out]
              }
            }
            n136 = property on="Camera Handle" class="DigNum (strict)"() -> ("Value"=w232:u32)  [unwired: 2 in, 2 out]
            n137 = call <vilib>:"MEPU-Acquisition-SetStreamState.vi"("hCamera IN"=w232, "uStreamState IN"=w242, "Error IN"=w238) -> ("hCamera OUT"=w241:u32, "Error OUT"=w240:errorcluster)  [unwired: 11 in]
            n138 = call "Get Buffer Size.vi"("phCamera IN"=w241, "Error IN"=w240) -> ("phCamera OUT"=w246:u32, "uBufferSize OUT"=w244:u32, "uWidth OUT"=w235:u32, "uHeight OUT"=w234:u32, "Error OUT"=w245:errorcluster)  [unwired: 8 in, 1 out]
            n139 = call <vilib>:"MEPU-Acquisition-GetNextFrame.vi"("hCamera IN"=w246, "Mode IN"=enum16{"UseArray", "UsePointer"}."UseArray", "uBufferSize IN"=w244, "Error IN"=w245) -> ("Data OUT"=w237:u8[], "pDescriptor"=w233:T9, "Error OUT"=w236:errorcluster)  [unwired: 7 in, 2 out]
            n140 = property on="Error OUT 2" class="Clust (strict)"("Value"=w236) -> ()  [unwired: 2 in, 2 out]
            n141 = case shown="No Error" w236 {
              tunnel: w237 -> [w250 _]
              tunnel: w235 -> [w249 _]
              tunnel: w234 -> [w248 _]
              tunnel: w233 -> [w247 _]
              frame No Error {
                n142 = property on="Save Data" class="Bool (strict)"() -> ("Value"=w251:bool)  [unwired: 2 in, 2 out]
                n143 = Type Cast(type=u16[] [] ("Data OUT"), x=w250) -> (*(type *) &x=w252:u16[])
                n144 = stacked-sequence {
                  seq-local: [_ w262 _] -> [_ _ w283]
                  seq-local: [w255 _ _] -> [_ _ w281]
                  tunnel: w252 -> [w260 _ _]
                  tunnel: w251 -> [_ w261 w282]
                  tunnel: w249 -> [w258 _ _]
                  tunnel: w248 -> [w257 _ _]
                  tunnel: w247 -> [_ _ _]
                  frame #0 {
                    n145 = Reshape Array(w260, w257, w258) -> (w255:u16[][])
                    n146 = local read "Div"() -> (w256:dbl)
                    n147 = property on="Waiting for Trigger" class="Bool (strict)"("Value"=FALSE ("Waiting for Trigger")) -> ()  [unwired: 2 in, 2 out]
                    n148 = Divide(x=w255, y=w256) -> (x/y=w254:dbl[][])
                    n149 = property on="Captured Image" class="IntGraph (strict)"("Value"=w254) -> ()  [unwired: 2 in, 2 out]
                  }
                  frame #1 {
                    n150 = case shown="True" w261 {
                      tunnel: [path "" ("File Path") w266] -> w262
                      frame False {
                      }
                      frame True {
                        n151 = property on="Racine chemin de sauvegarde" class="Path"() -> ("Value"=w264:path)  [unwired: 2 in, 2 out]
                        n152 = property on="Automatic\nfolder naming" class="Bool (strict)"() -> ("Value"=w265:bool)  [unwired: 2 in, 2 out]
                        n153 = case shown="False" w265 {
                          tunnel: [w267 w274] -> w266
                          tunnel: w264 -> [w273 w275]
                          frame False {
                            n154 = property on="Nom du fichier" class="Str"() -> ("Value"=w270:string)  [unwired: 2 in, 2 out]
                            n155 = property on="Indice" class="DigNum (strict)"() -> ("Value"=w269:u32)  [unwired: 2 in, 2 out]
                            n156 = property on="Overwrite?" class="Bool (strict)"() -> ("Value"=w268:bool)  [unwired: 2 in, 2 out]
                            n157 = call "CheckFolder.vi"("Overwrite?"=w268, "Index"=w269, "File Name"=w270, "Folder Path Control"=w273) -> ("Warning"=w271:bool, "Message"=w272:string, "File Path"=w267:path)  [unwired: 5 in]
                            n158 = property on="Message" class="Str"("Value"=w272) -> ()  [unwired: 2 in, 2 out]
                            n159 = property on="Warning" class="Bool (strict)"("Value"=w271) -> ()  [unwired: 2 in, 2 out]
                          }
                          frame True {
                            n160 = property on="Nom du fichier" class="Str"() -> ("Value"=w278:string)  [unwired: 2 in, 2 out]
                            n161 = property on="Indice" class="DigNum (strict)"() -> ("Value"=w279:u32)  [unwired: 2 in, 2 out]
                            n162 = property on="Overwrite?" class="Bool (strict)"() -> ("Value"=w280:bool)  [unwired: 2 in, 2 out]
                            n163 = call "CheckMonthDateFolder.vi"("Overwrite?"=w280, "Index"=w279, "File Name"=w278, "Folder Path Control"=w275) -> ("Warning"=w276:bool, "Message"=w277:string, "File Path"=w274:path)  [unwired: 5 in]
                            n164 = property on="Warning" class="Bool (strict)"("Value"=w276) -> ()  [unwired: 2 in, 2 out]
                            n165 = property on="Message" class="Str"("Value"=w277) -> ()  [unwired: 2 in, 2 out]
                          }
                        }
                      }
                    }
                  }
                  frame #2 {
                    n166 = case shown="True" w282 {
                      tunnel: w283 -> [_ w285]
                      tunnel: w281 -> [_ w284]
                      frame False {
                      }
                      frame True {
                        n167 = Not A Number/Path/Refnum?(number/path/refnum=w285) -> (NaN/Path/Refnum?=w286:bool)
                        n168 = case shown="False" w286 {
                          tunnel: w285 -> [w290 _]
                          tunnel: w284 -> [w292 _]
                          frame False {
                            # "Save Image\nand data"
                            n169 = call "SavePicture.vi"("File Path"=w290, "Image Pixels (U16)"=w292) -> ("error out"=w298:errorcluster)  [unwired: 9 in]
                            n170 = property on="Nom du fichier" class="Str"() -> ("Value"=w289:string)  [unwired: 2 in, 2 out]
                            n171 = property on="Indice" class="DigNum (strict)"() -> ("Value"=w288:u32)  [unwired: 2 in, 2 out]
                            n172 = property on="Exposure Time" class="Slide (strict)"() -> ("Value"=w287:dbl)  [unwired: 2 in, 2 out]
                            n173 = Unbundle By Name(w298) -> ("source"=w295:string, "status"=w296:bool)
                            n174 = call "FindLineAndOverwrite_Double.vi"("Exposure path"=w290, "Name"=w289, "Index"=w288, "Exposure"=w287) -> ("error out"=w291:errorcluster)  [unwired: 11 in]
                            n175 = Unbundle By Name(w291) -> ("status"=w297:bool, "source"=w299:string)
                            n176 = Or(x=w296, y=w297) -> (x .or. y?=w294:bool)
                            n177 = case shown="False" w294 {
                              tunnel: w299 -> [_ w303]
                              tunnel: w295 -> [_ w306]
                              tunnel: "\r\n" -> [_ w304]
                              frame False {
                                n178 = property on="Mode de Sauvegarde" class="Ring (strict)"() -> ("Value"=w301:u16)  [unwired: 2 in, 2 out]
                                n179 = property on="Indice" class="DigNum (strict)"() -> ("Value"=w302:u32)  [unwired: 2 in, 2 out]
                                n180 = Add(x=w302, y=w301) -> (x+y=w300:u32)
                                n181 = property on="Indice" class="DigNum (strict)"("Value"=w300) -> ()  [unwired: 2 in, 2 out]
                              }
                              frame True {
                                n182 = Concatenate Strings(w306, w304, w303) -> (w305:string)
                                n183 = property on="Message" class="Str"("Value"=w305) -> ()  [unwired: 2 in, 2 out]
                              }
                            }
                          }
                          frame True {
                          }
                        }
                      }
                    }
                  }
                }
              }
              frame Error {
              }
            }
          }
          event "Bind Path to Camera": Value Change {
            n184 = event-data() -> ()  [unwired: 1 in, 6 out]
            n185 = property on="Imager" class="Ring (strict)"() -> ("StringsAndValues[]"=w314:T7)  [unwired: 2 in, 2 out]
            n186 = for {
              tunnel: w314 -> [w322] mode=indexing
              tunnel: [w317] -> w313 mode=indexing
              i -> [w318]
              n187 = Unbundle By Name(w322) -> ("String"=w321:string)
              n188 = Concatenate Strings("Choose path to save data\nfrom ", w321) -> (w319:string)
              n189 = Two Button Dialog(message=w319) -> (T button?=w317:bool)  [unwired: 2 in]
              n190 = case shown="True" w317 {
                tunnel: w318 -> [_ w324]
                frame False {
                }
                frame True {
                  n191 = call "File Dialog"() -> ("selected path"=w325:path, "error out"=w323:errorcluster)  [unwired: 12 in, 2 out]
                  n192 = case shown="No Error" w323 {
                    tunnel: w325 -> [w330 _]
                    tunnel: w324 -> [w327 _]
                    frame No Error {
                      n193 = property on="Chemins\n de sauvegarde" class="Arr (strict)"() -> ("Value"=w331:path[])  [unwired: 2 in, 2 out]
                      n194 = Array Size(array=w331) -> (size(s)=w329:i32)
                      n195 = Less Or Equal?(x=w329, y=w327) -> (x <= y?=w328:bool)
                      n196 = case shown="False" w328 {
                        tunnel: w331 -> [w335 w339]
                        tunnel: w330 -> [w333 w337]
                        tunnel: w327 -> [w334 w338]
                        tunnel: [w332 w336] -> w326
                        frame False {
                          n197 = Replace Array Subset(array=w335, new element=w333, index=w334) -> (w332:path[])
                        }
                        frame True {
                          n198 = Insert Into Array(array=w339, index=w338, new element=w337) -> (w336:path[])
                        }
                      }
                      n199 = property on="Chemins\n de sauvegarde" class="Arr (strict)"("Value"=w326) -> ()  [unwired: 2 in, 2 out]
                    }
                    frame Error {
                    }
                  }
                }
              }
            }
            n200 = property on="Imager" class="Ring (strict)"() -> ("Value"=w311:u32)  [unwired: 2 in, 2 out]
            n201 = property on="Imager Serial #" class="Arr (strict)"() -> ("Value"=w310:u32[])  [unwired: 2 in, 2 out]
            n202 = Search 1D Array(1D array=w310, element=w311) -> (index of element=w309:i32)  [unwired: 1 in]
            n203 = Index Array(array=w313, index=w309) -> (element=w312:bool)
            n204 = case shown="True" w312 {
              frame False {
              }
              frame True {
                # "If path to current cam data was changed, update on interface"
                n205 = property on="Chemins\n de sauvegarde" class="Arr (strict)"() -> ("Value"=w316:path[])  [unwired: 2 in, 2 out]
                n206 = Index Array(array=w316) -> (element=w315:path)  [unwired: 1 in]
                n207 = property on="Racine chemin de sauvegarde" class="Path"("Value"=w315) -> ()  [unwired: 2 in, 2 out]
              }
            }
          }
          event "Snap current Data": Value Change {
            n208 = event-data() -> ()  [unwired: 1 in, 6 out]
            n209 = stacked-sequence {
              seq-local: [w347 _] -> [_ w363]
              frame #0 {
                n210 = property on="Racine chemin de sauvegarde" class="Path"() -> ("Value"=w343:path)  [unwired: 2 in, 2 out]
                n211 = property on="Nom du fichier" class="Str"() -> ("Value"=w344:string)  [unwired: 2 in, 2 out]
                n212 = property on="Indice" class="DigNum (strict)"() -> ("Value"=w345:u32)  [unwired: 2 in, 2 out]
                n213 = property on="Overwrite?" class="Bool (strict)"() -> ("Value"=w346:bool)  [unwired: 2 in, 2 out]
                n214 = property on="Automatic\nfolder naming" class="Bool (strict)"() -> ("Value"=w340:bool)  [unwired: 2 in, 2 out]
                n215 = case shown="False" w340 {
                  tunnel: [w350 w361] -> w347
                  tunnel: w346 -> [w351 w360]
                  tunnel: w345 -> [w352 w359]
                  tunnel: w344 -> [w353 w358]
                  tunnel: w343 -> [w354 w357]
                  tunnel: [w349 w356] -> w342
                  tunnel: [w348 w355] -> w341
                  frame False {
                    n216 = call "CheckFolder.vi"("Overwrite?"=w351, "Index"=w352, "File Name"=w353, "Folder Path Control"=w354) -> ("Warning"=w348:bool, "Message"=w349:string, "File Path"=w350:path)  [unwired: 5 in]
                  }
                  frame True {
                    n217 = call "CheckMonthDateFolder.vi"("Overwrite?"=w360, "Index"=w359, "File Name"=w358, "Folder Path Control"=w357) -> ("Warning"=w355:bool, "Message"=w356:string, "File Path"=w361:path)  [unwired: 5 in]
                  }
                }
                n218 = property on="Warning" class="Bool (strict)"("Value"=w341) -> ()  [unwired: 2 in, 2 out]
                n219 = property on="Message" class="Str"("Value"=w342) -> ()  [unwired: 2 in, 2 out]
              }
              frame #1 {
                n220 = Not A Number/Path/Refnum?(number/path/refnum=w363) -> (NaN/Path/Refnum?=w362:bool)
                n221 = case shown="False" w362 {
                  tunnel: w363 -> [w368 _]
                  frame False {
                    # "Save Image\nand data"
                    n222 = property on="Captured Image" class="IntGraph (strict)"() -> ("Value"=w369:dbl[][])  [unwired: 2 in, 2 out]
                    n223 = call "SavePicture.vi"("File Path"=w368, "Image Pixels (U16)"=w369) -> ("error out"=w375:errorcluster)  [unwired: 9 in]
                    n224 = property on="Nom du fichier" class="Str"() -> ("Value"=w367:string)  [unwired: 2 in, 2 out]
                    n225 = property on="Indice" class="DigNum (strict)"() -> ("Value"=w366:u32)  [unwired: 2 in, 2 out]
                    n226 = property on="Exposure Time" class="Slide (strict)"() -> ("Value"=w365:dbl)  [unwired: 2 in, 2 out]
                    n227 = Unbundle By Name(w375) -> ("source"=w372:string, "status"=w373:bool)
                    n228 = call "FindLineAndOverwrite_Double.vi"("Exposure path"=w368, "Name"=w367, "Index"=w366, "Exposure"=w365) -> ("error out"=w364:errorcluster)  [unwired: 11 in]
                    n229 = Unbundle By Name(w364) -> ("status"=w374:bool, "source"=w376:string)
                    n230 = Or(x=w373, y=w374) -> (x .or. y?=w371:bool)
                    n231 = case shown="False" w371 {
                      tunnel: w376 -> [_ w380]
                      tunnel: w372 -> [_ w383]
                      tunnel: "\r\n" -> [_ w381]
                      frame False {
                        n232 = property on="Mode de Sauvegarde" class="Ring (strict)"() -> ("Value"=w378:u16)  [unwired: 2 in, 2 out]
                        n233 = property on="Indice" class="DigNum (strict)"() -> ("Value"=w379:u32)  [unwired: 2 in, 2 out]
                        n234 = Add(x=w379, y=w378) -> (x+y=w377:u32)
                        n235 = property on="Indice" class="DigNum (strict)"("Value"=w377) -> ()  [unwired: 2 in, 2 out]
                      }
                      frame True {
                        n236 = Concatenate Strings(w383, w381, w380) -> (w382:string)
                        n237 = property on="Message" class="Str"("Value"=w382) -> ()  [unwired: 2 in, 2 out]
                      }
                    }
                  }
                  frame True {
                  }
                }
              }
            }
          }
        }
      }
      n238 = property on="Error OUT" class="Clust (strict)"("Value"=w69) -> ()  [unwired: 2 in, 2 out]
    }
    frame #4 {
      w386 = T1 2 items=["START_STREAM", "PAUSE_STREAM", "STOP_STREAM"] ("uStreamState IN")
      # "Ignore errors here to ensure as\ncomplete a clean up as possible."
      n239 = property on="Camera Handle" class="DigNum (strict)"() -> ("Value"=w384:u32)  [unwired: 2 in, 2 out]
      n240 = call <vilib>:"MEPU-Acquisition-SetStreamState.vi"("hCamera IN"=w384, "uStreamState IN"=w386) -> ("hCamera OUT"=w388:u32)  [unwired: 12 in, 1 out]
      n241 = call <vilib>:"MEPU-Initialization-Uninitialize.vi"("hCamera IN"=w388) -> ("Error OUT"=w387:errorcluster)  [unwired: 14 in]
      n242 = stacked-sequence {
        tunnel: w387 -> [_]
        frame #0 {
          n243 = call <vilib>:"MEPU-Initialization-UninitializeSystem.vi"() -> ()  [unwired: 15 in, 1 out]
        }
      }
    }
  }
  n244 = Or(x=w3, y=w2) -> (x .or. y?=w1:bool)
  n245 = property on="stop" class="Bool (strict)"("Value"=w1) -> ()  [unwired: 2 in, 2 out]
